vi "New Field UI.vi"() -> (2 "Cancelled":bool, 3 "Field":refnum<class "Type.lvclass">)   [LabVIEW 2020, in "Conditum-Tools.lvlib" / "Entity Editor.lvclass"]
uses:
  Entity Editor.lvclass
  Conditum-Clone/Columns/Type/Type.lvclass
  Conditum-Clone/Columns/Type/Type.lvclass/Type.ctl
  ColumnPanel/ColumnPanel.lvclass
  C:/Program Files (x86)/National Instruments/LabVIEW 2020/vi.lib/IlluminatedG/IG OOPanel/OOPanel/Panel/Panel.lvclass
  <vilib>/IlluminatedG/IG OOPanel/OOPanel/Manager/Manager.lvclass
  <vilib>/Utility/LVClass/Get LV Class Name.vi
  Conditum-Tools.lvlib
panel:
  in  "Cancel":bool
  in  "OK":bool
  in  "Field Type":i32(listbox)
  # "Select a field type:"
  # "Set the initial field configuration, this can be also changed after creation:"
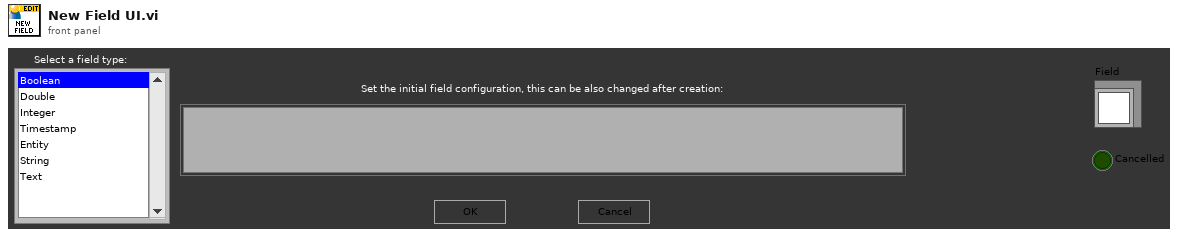
[diagram p1: front panel]
types:
  T1 = enum8{"Enabled", "Disabled", "Disabled and Grayed Out"}
  T2 = typedef "Conditu2.lvlib/Field Type.ctl" = enum16{"None", "ID", "Boolean", "Integer", "Double", "Timestamp", "String", "Text", "Entity"}
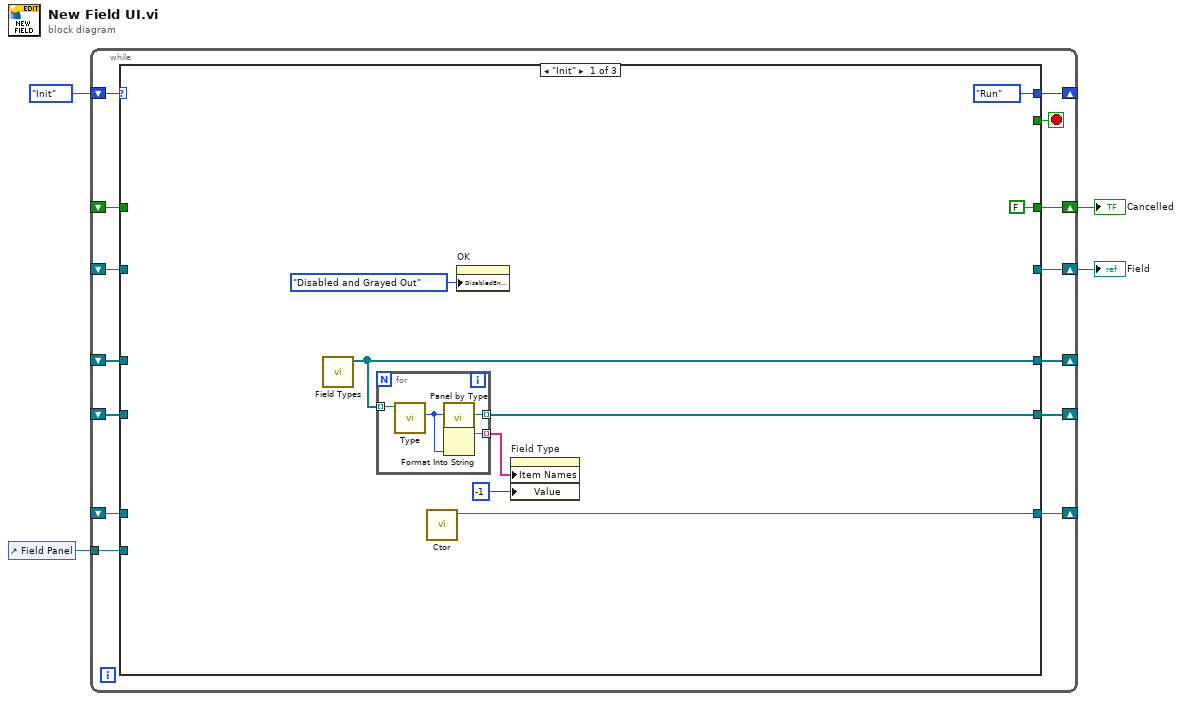
[diagram p0: block diagram]
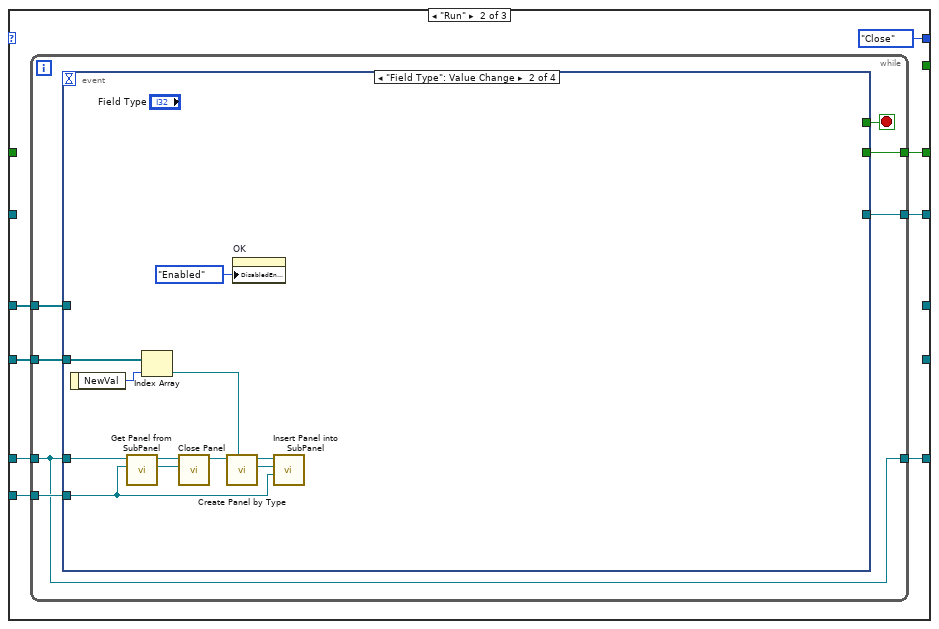
[diagram p2: hidden frame]
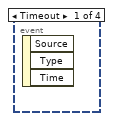
[diagram p3: hidden frame]
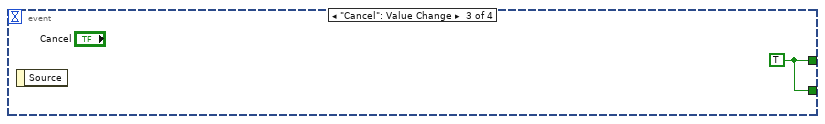
[diagram p4: hidden frame]
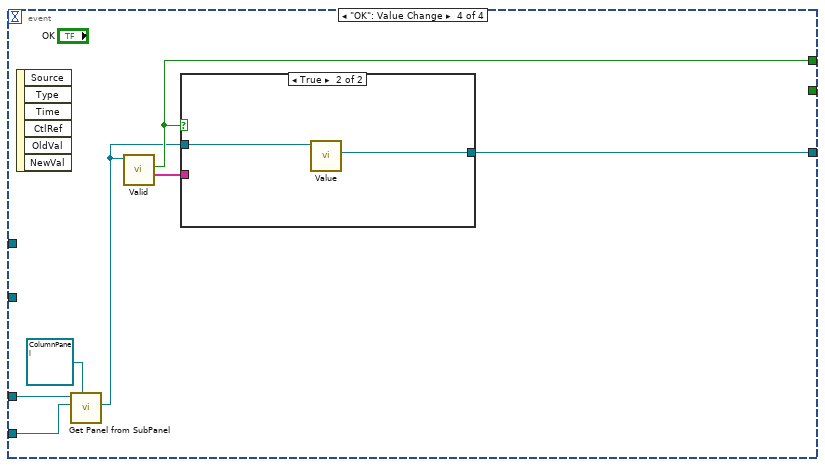
[diagram p5: hidden frame]
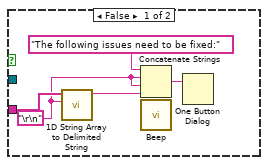
[diagram p6: hidden frame]
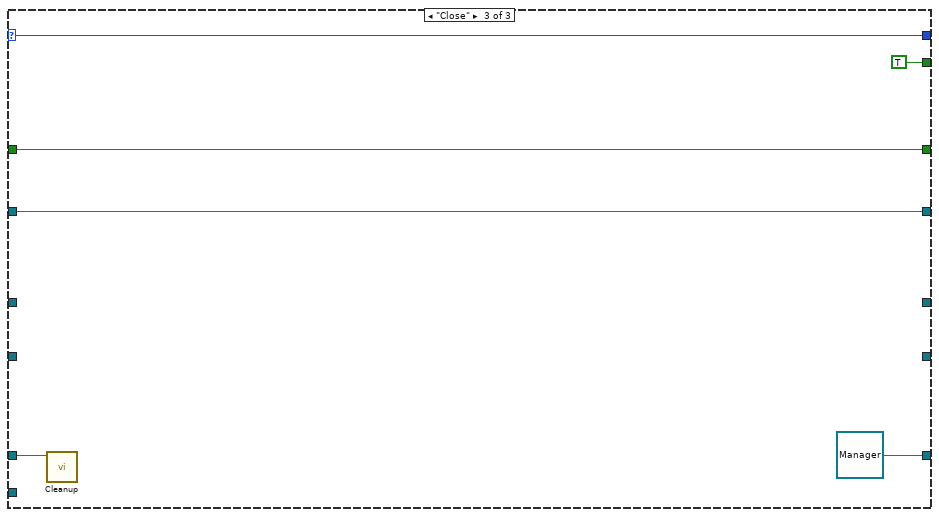
[diagram p7: hidden frame]
diagram:
  n1 = control-ref of="Field Panel"() -> (w2:refnum<vi>)
  n2 = while {
    shift-right: [w17] -> _
    shift-left: enum16{"Init", "Run", "Close"}."Init" ("Basic UI State") -> [w18]
    shift-right: [w15] -> w3
    shift-left: _ -> [w14]
    shift-right: [w13] -> _
    shift-left: _ -> [w12]
    shift-right: [w11] -> _
    shift-left: _ -> [w10]
    shift-right: [w9] -> _
    shift-left: _ -> [w8]
    tunnel: w2 -> [w7]
    shift-right: [w6] -> w1
    shift-left: _ -> [w5]
    stop <- w16 stop-if-true
    n3 = case shown="\"Init\"" w18 {
      selector: w18 -> [_ _ w77]
      tunnel: [enum16{"Init", "Run", "Close"}."Run" ("Basic UI State") enum16{"Init", "Run", "Close"}."Close" ("Basic UI State") w77] -> w17
      tunnel: [_ _ TRUE] -> w16
      tunnel: [FALSE w35 w75] -> w15
      tunnel: w14 -> [_ _ w75]
      tunnel: [w24 _ _] -> w13
      tunnel: w12 -> [_ w37 _]
      tunnel: [w23 _ _] -> w11
      tunnel: w10 -> [_ w36 _]
      tunnel: [w21 w33 refnum<class "Manager.lvclass"> refnum ("Manager out")] -> w9
      tunnel: w8 -> [_ w34 w74]
      tunnel: w7 -> [_ w32 _]
      tunnel: [_ w31 w72] -> w6
      tunnel: w5 -> [_ _ w72]
      frame "Init" {
        n4 = call "Field Types.vi"() -> ("Creatable Field Types"=w24:refnum<class "Type.lvclass">[])  [unwired: 11 in]
        n5 = for {
          tunnel: w24 -> [w30] mode=indexing
          tunnel: [w29] -> w23 mode=indexing
          tunnel: [w27] -> w22 mode=indexing
          n6 = call "Type.vi"("Type in"=w30) -> ("Type"=w28:T2)  [unwired: 10 in]
          n7 = call "Panel by Type.vi"("Type"=w28) -> ("ColumnPanel"=w29:refnum<class "ColumnPanel.lvclass">)  [unwired: 10 in]
          n8 = Format Into String(w28) -> (resulting string=w27:string)  [unwired: 3 in, 1 out]
        }
        n9 = call <vilib>:"Ctor.vi"() -> ("Manager out"=w21:refnum<class "Manager.lvclass">)  [unwired: 10 in, 1 out]
        n10 = property on="OK" class="Bool"("DisabledEnum"=T1."Disabled and Grayed Out" ("Disabled")) -> ()  [unwired: 2 in, 2 out]
        n11 = property on="Field Type" class="LstBox (strict)"("Item Names"=w22, "Value"=-1 ("Field Type")) -> ()  [unwired: 2 in, 2 out]
      }
      frame "Run" {
        n12 = while {
          tunnel: w37 -> [w45]
          tunnel: w36 -> [w44]
          tunnel: [w42] -> w35
          tunnel: w34 -> [w40]
          tunnel: [w40] -> w33
          tunnel: w32 -> [w41]
          tunnel: [w39] -> w31
          stop <- w43 stop-if-true
          n13 = event shown="[1] \"Field Type\": Value Change" {
            selector: _ -> [_ _ _ _]
            dyn-events: _ -> [_ _ _ _]
            timeout: _ -> [_ _ _ _]
            tunnel: w45 -> [_ _ _ _]
            tunnel: w44 -> [_ w56 _ _]
            tunnel: [_ _ w57 w60] -> w43
            tunnel: [_ _ w57 _] -> w42
            tunnel: w40 -> [_ w52 _ w64]
            tunnel: w41 -> [_ w50 _ w63]
            tunnel: [_ _ _ w58] -> w39
            event Timeout {
              n14 = event-data() -> ()  [unwired: 1 in, 3 out]
            }
            event "Field Type": Value Change {
              n15 = event-data() -> ("NewVal"=w55:i32)  [unwired: 1 in]
              n16 = call <vilib>:"Get Panel from SubPanel.vi"("SubPanel"=w50, "Manager in"=w52) -> ("Panel"=w46:refnum<class "Panel.lvclass">, "Manager out"=w48:refnum<class "Manager.lvclass">)  [unwired: 6 in, 2 out]
              n17 = Index Array(array=w56, index=w55) -> (element=w54:refnum<class "ColumnPanel.lvclass">)
              n18 = call <vilib>:"Close Panel.vi"("Panel"=w46, "Manager in"=w48) -> ("Manager out"=w47:refnum<class "Manager.lvclass">)  [unwired: 8 in, 1 out]
              n19 = call <vilib>:"Create Panel by Type.vi"("Panel Type"=w54, "Manager in"=w47) -> ("Panel"=w51:refnum<class "ColumnPanel.lvclass">, "Manager out"=w53:refnum<class "Manager.lvclass">)  [unwired: 7 in, 1 out]
              n20 = property on="OK" class="Bool"("DisabledEnum"=T1."Enabled" ("Disabled")) -> ()  [unwired: 2 in, 2 out]
              n21 = call <vilib>:"Insert Panel into SubPanel.vi"("SubPanel"=w50, "Panel In"=w51, "Manager in"=w53) -> ()  [unwired: 6 in, 3 out]
            }
            event "Cancel": Value Change {
              w57 = TRUE
              n22 = event-data() -> ()  [unwired: 1 in, 1 out]
            }
            event "OK": Value Change {
              n23 = event-data() -> ()  [unwired: 1 in, 6 out]
              n24 = call <vilib>:"Get Panel from SubPanel.vi"("Panel Type (Panel)"=refnum<class "ColumnPanel.lvclass"> refnum ("Conditum-Tools.lvlib:ColumnPanel.lvclass"), "SubPanel"=w63, "Manager in"=w64) -> ("Panel"=w59:refnum<class "ColumnPanel.lvclass">)  [unwired: 5 in, 3 out]
              n25 = call "Valid.vi"("ColumnPanel in"=w59) -> ("Issues"=w61:string[], "Valid?"=w60:bool)  [unwired: 8 in, 1 out]
              n26 = case shown="True" w60 {
                tunnel: w61 -> [w69 _]
                tunnel: w59 -> [_ w71]
                tunnel: [_ w70] -> w58
                frame False {
                  w65 = "\r\n"
                  n27 = call <vilib>:"1D String Array to Delimited String.vi"("delimiter"=w65, "string array"=w69) -> ("delimited string"=w66:string)  [unwired: 9 in]
                  n28 = Concatenate Strings("The following issues need to be fixed:", w65, w65, w66) -> (w67:string)
                  n29 = call <vilib>:"Beep.vi"() -> ()  [unwired: 12 in]
                  n30 = One Button Dialog(message=w67) -> ()  [unwired: 1 in, 1 out]
                }
                frame True {
                  n31 = call "Value.vi"("ColumnPanel in"=w71) -> ("Type Value"=w70:refnum<class "Type.lvclass">)  [unwired: 9 in, 1 out]
                }
              }
            }
          }
        }
      }
      frame "Close" {
        n32 = call <vilib>:"Cleanup.vi"("Manager in"=w74) -> ()  [unwired: 8 in, 3 out]
      }
    }
  }
  "Cancelled" <- w3
  "Field" <- w1
